vi "pb_inst_pbonly.vi"(8 "error in (no error)":errorcluster, 10 "PB Instruction":T1={"Instruct Data"=0, "Op Code"=0, "Flags"=[FALSE, FALSE, FALSE, FALSE, FALSE, FALSE, FALSE, FALSE, FALSE, FALSE, FALSE, FALSE, FALSE, FALSE, FALSE, FALSE, FALSE, FALSE, FALSE, FALSE, FALSE, FALSE, FALSE, FALSE], "Comments"="", "Time"=0.016675} {"Time" format="%.3p"; "Op Code" items=["Continue", "Stop", "Loop", "End Loop", "JSR", "RTS", "Branch", "Long Delay", "Wait"]}, 11 "path in":path=path "C:/Program Files/SpinCore/SpinAPI/dll/spinapi.dll") -> (0 "error out":errorcluster, 3 "path out":path)   [LabVIEW 2012]
panel:
  # "1"
  # "2"
  # "3"
  # "4"
  # "5"
  # "6"
  # "7"
  # "8"
  # "9"
  # "10"
  # "11"
  # "12"
  # "13"
  # "14"
  # "15"
  # "16"
  # "17"
  # "18"
  # "19"
  # "20"
  # "21"
  # "22"
  # "23"
  # "24"
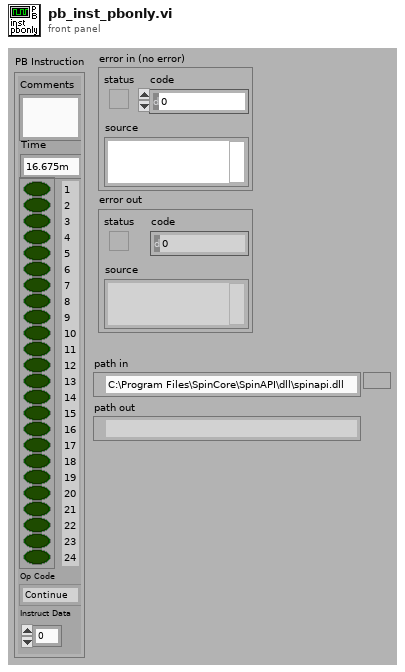
[diagram p1: front panel]
types:
  T1 = cluster{"Instruct Data":i32, "Op Code":i32, "Flags":bool[], "Comments":string, "Time":dbl}
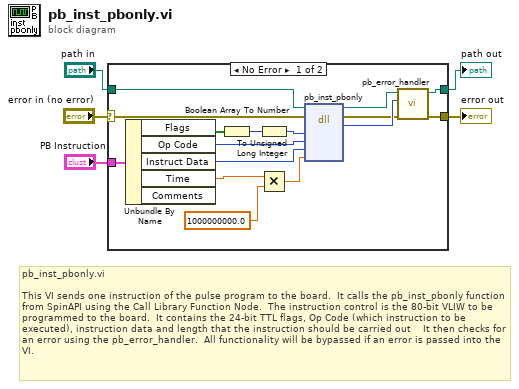
[diagram p0: block diagram]
diagram:
  # "pb_inst_pbonly.vi\n\nThis VI sends one instruction of the pulse program to the board.  It calls the pb_inst_pbonly function from SpinAPI using the Call Library Function Node.  The instruction control is the 80-bit VLIW to be programmed to the board.  It contains the 24-bit TTL flags, Op Code (which instruction to be executed), instruction data and length that the instruction should be carried out    It then checks for an error using the pb_error_handler.  All functionality will be bypassed if an error is passed into the VI."
  n1 = case shown="No Error" "error in (no error)" {
    selector: "error in (no error)" -> [w11 w23]
    tunnel: "PB Instruction" -> [w21 _]
    tunnel: [w6 w23] -> w4
    tunnel: "path in" -> [w10 w22]
    tunnel: [w7 w22] -> w1
    frame No Error {
      n2 = Unbundle By Name(w21) -> ("Flags"=w20:bool[], "Op Code"=w17:i32, "Instruct Data"=w16:i32, "Time"=w14:dbl)  [unwired: 1 out]
      n3 = Boolean Array To Number(Boolean array=w20) -> (number=w19:u32)
      n4 = To Unsigned Long Integer(number=w19) -> (unsigned 32bit integer=w18:u32)
      n5 = Multiply(x=w14, y=1000000000.0) -> (x*y=w12:dbl)
      n6 = dll-call lib="C:/Program Files/SpinCore/SpinAPI/dll/spinapi.dll" fn="pb_inst_pbonly"(path in=w10, error in=w11, "flags"=w18, "inst"=w17, "inst_data"=w16, "length"=w12) -> (path out=w9:path, error out=w8:errorcluster, "return type"=w15:i32)  [unwired: 5 in]
      n7 = call "pb_error_handler.vi"("error in (no error)"=w8, "return code"=w15, "path in"=w9) -> ("error out"=w6:errorcluster, "path out"=w7:path)  [unwired: 7 out]
    }
    frame Error {
    }
  }
  "error out" <- w4
  "path out" <- w1
